vi "SNAFU to Decimal.vi"(1 "SNAFU Number":string) -> (0 "Decimal Number":i64)   [LabVIEW 2020, in "AoC 2022.lvlib"]
uses:
  AoC 2022.lvlib
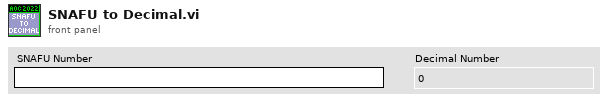
[diagram p1: front panel]
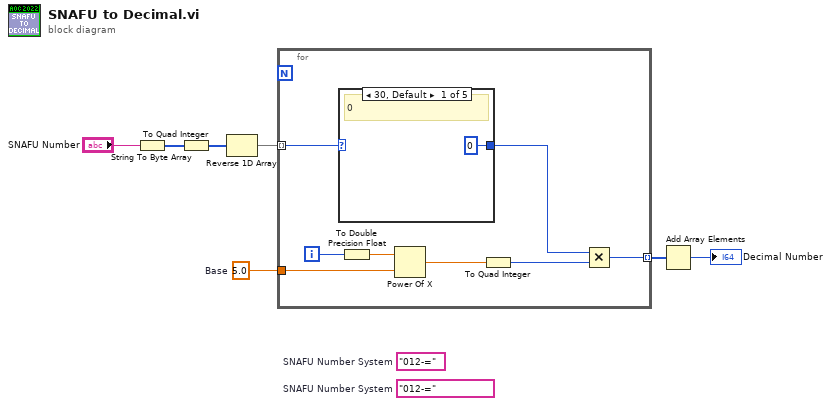
[diagram p0: block diagram]
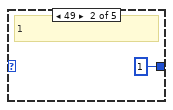
[diagram p2: hidden frame]
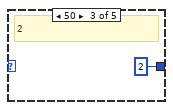
[diagram p3: hidden frame]
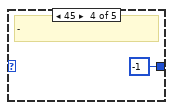
[diagram p4: hidden frame]
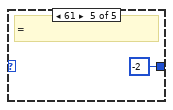
[diagram p5: hidden frame]
diagram:
  (unwired) "012-="  # SNAFU Number System
  (unwired) "012-="  # SNAFU Number System
  w7 = 5.0  # Base
  n1 = String To Byte Array(string="SNAFU Number") -> (unsigned byte array=w2:u8[])
  n2 = To Quad Integer(1:w2) -> (0:w4:i64[])
  n3 = Reverse 1D Array(array=w4) -> (reversed array=w3:i64[])
  n4 = for {
    tunnel: w3 -> [w14] mode=indexing
    tunnel: w7 -> [w11]
    tunnel: [w15] -> w5 mode=indexing
    i -> [w12]
    n5 = case shown="30, Default" w14 {
      tunnel: [i64 0 i64 1 i64 2 i64 -1 i64 -2] -> w13
      frame 48, Default {
        # "0"
      }
      frame 49 {
        # "1"
      }
      frame 50 {
        # "2"
      }
      frame 45 {
        # "-"
      }
      frame 61 {
        # "="
      }
    }
    n6 = To Double Precision Float(number=w12) -> (double precision float=w8:dbl)
    n7 = Power Of X(1:w11, 2:w8) -> (0:w10:dbl)
    n8 = To Quad Integer(1:w10) -> (0:w9:i64)
    n9 = Multiply(x=w13, y=w9) -> (x*y=w15:i64)
  }
  n10 = Add Array Elements(numeric array=w5) -> (sum=→"Decimal Number":i64)
